vi "AB_Engine_Update_Paths_In_Palette_File.vi"(0 "old palette path":path, 1 "new palette path":path, 2 "old paths":path[](array[path]), 3 "new paths":path[](array[path]), 4 "old dir paths":path[](array[path]), 5 "new dir paths":path[](array[path]), 6 "application reference":refnum<vi>, 7 "error in":errorcluster) -> (19 "error out":errorcluster)   [LabVIEW 2020]
uses:
  <vilib>/Palette API/Palette Menu/Public Type Define/Palette Data.ctl
  <vilib>/Palette API/Palette Menu/Public Type Define/View Format.ctl
  <vilib>/Palette API/Palette Menu/Public Type Define/Items.ctl
  <vilib>/Palette API/Palette Menu/Public Type Define/Item.ctl
  <vilib>/Palette API/Palette Menu/Public Type Define/Help Info.ctl
  <vilib>/Palette API/Palette Menu/Public Type Define/Synchronize Info.ctl
  <vilib>/Palette API/Palette Menu/Public Type Define/Palette type.ctl
  <vilib>/Palette API/Palette Menu/Palette Menu.lvlib
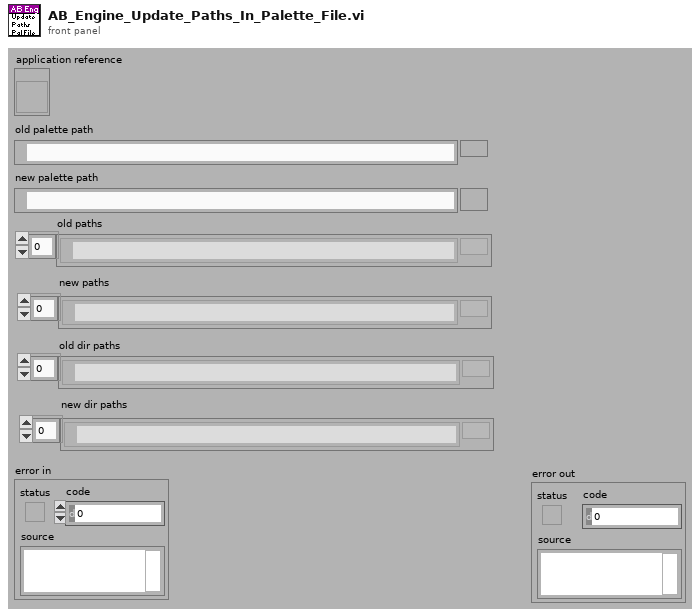
[diagram p1: front panel]
types:
  T1 = typedef "Palette Menu.lvlib/Palette Data.ctl" = cluster{"display name":string, "view format":T2, "palette width":i16, "items":T3, "256 color icon":picture, "B&W color icon":picture, "help information":T5, "palette description":string, "synchronize information":T6}
  T2 = typedef "Palette Menu.lvlib/View Format.ctl" = u16
  T3 = typedef "Palette Menu.lvlib/Items.ctl" = T4[]
  T4 = typedef "Palette Menu.lvlib/Item.ctl" = cluster{"item path":path, "library path":path, "use default lvlib palette":bool, "short name":string, "place VI contents":bool, "hide synchronized item":bool, "reserve spot for synch item":bool, "configure when placing VI contents":bool}
  T5 = typedef "Palette Menu.lvlib/Help Info.ctl" = cluster{"help tag":string, "help file path ":path}
  T6 = typedef "Palette Menu.lvlib/Synchronize Info.ctl" = cluster{"synchronize with directory":bool, "synchronize directory path":path}
  T7 = typedef "Palette Menu.lvlib/Palette type.ctl" = i32
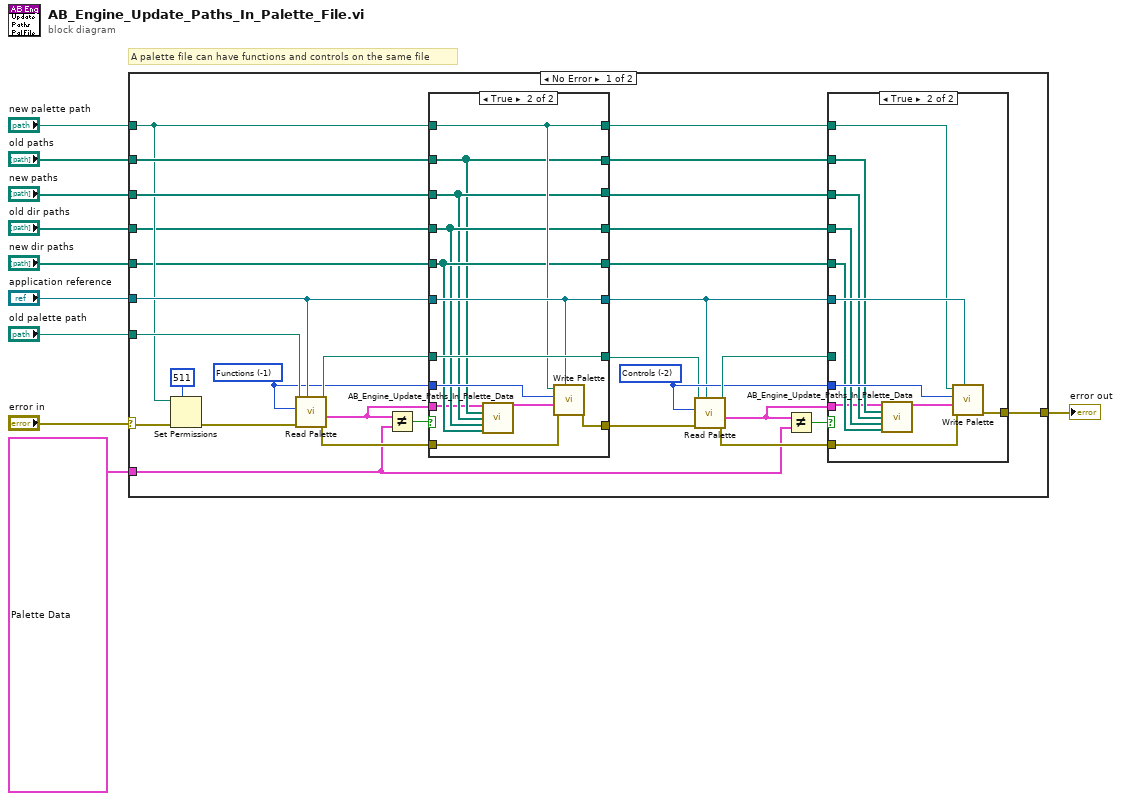
[diagram p0: block diagram]
diagram:
  # "A palette file can have functions and controls on the same file"
  n1 = case shown="No Error" "error in" {
    selector: "error in" -> [w18 w73]
    tunnel: "new palette path" -> [w15 _]
    tunnel: "old paths" -> [w35 _]
    tunnel: "new paths" -> [w34 _]
    tunnel: "application reference" -> [w33 _]
    tunnel: "old palette path" -> [w40 _]
    tunnel: [w19 w73] -> w4
    tunnel: T1 {"display name"="", "view format"=2, "palette width"=0, "items"=[], "256 color icon"=bytes[0], "B&W color icon"=bytes[0], "help information"={"help tag"="", "help file path "=path ""}, "palette description"="", "synchronize information"={"synchronize with directory"=FALSE, "synchronize directory path"=path ""}} ("palette data") -> [w20 _]
    tunnel: "old dir paths" -> [w14 _]
    tunnel: "new dir paths" -> [w13 _]
    frame No Error {
      w27 = T7 -2 items=["Functions"=-1, "Controls"=-2] ("palette type")
      w32 = T7 -1 items=["Functions"=-1, "Controls"=-2] ("palette type")
      n2 = Set Permissions(7:i16 511 ("permissions"), 8:w18, 11:w15) -> (0:w17:errorcluster)  [unwired: 2 in, 1 out]
      n3 = call <vilib>:"Read Palette.vi"("application reference"=w33, "error in (no error)"=w17, "palette type"=w32, "palette path"=w40) -> ("error out"=w38:errorcluster, "palette data"=w36:T1, "duplicate palette path"=w37:path)  [unwired: 5 in]
      n4 = Not Equal?(x=w36, y=w20) -> (x != y?=w39:bool)
      n5 = case shown="True" w39 {
        tunnel: w38 -> [w55 w71]
        tunnel: w37 -> [w56 w69]
        tunnel: w36 -> [_ w62]
        tunnel: w15 -> [w60 w67]
        tunnel: w35 -> [w59 w63]
        tunnel: w34 -> [w58 w64]
        tunnel: w33 -> [w57 w68]
        tunnel: w32 -> [_ w72]
        tunnel: [w55 w70] -> w26
        tunnel: [w56 w69] -> w25
        tunnel: [w57 w68] -> w24
        tunnel: [w58 w64] -> w23
        tunnel: [w59 w63] -> w22
        tunnel: [w60 w67] -> w21
        tunnel: [w54 w65] -> w12
        tunnel: w14 -> [w54 w65]
        tunnel: [w53 w66] -> w11
        tunnel: w13 -> [w53 w66]
        frame False {
        }
        frame True {
          n6 = call <vilib>:"AB_Engine_Update_Paths_In_Palette_Data.vi"("palette data in"=w62, "old paths"=w63, "new paths"=w64, "old dir paths"=w65, "new dir paths"=w66) -> ("palette data out"=w61:T1)  [unwired: 10 in]
          n7 = call <vilib>:"Write Palette.vi"("application reference"=w68, "error in (no error)"=w71, "palette data"=w61, "palette type"=w72, "palette path"=w67) -> ("error out"=w70:errorcluster)  [unwired: 6 in]
        }
      }
      n8 = call <vilib>:"Read Palette.vi"("application reference"=w24, "error in (no error)"=w26, "palette type"=w27, "palette path"=w25) -> ("error out"=w30:errorcluster, "palette data"=w28:T1, "duplicate palette path"=w29:path)  [unwired: 5 in]
      n9 = Not Equal?(x=w28, y=w20) -> (x != y?=w31:bool)
      n10 = case shown="True" w31 {
        tunnel: w30 -> [w41 w51]
        tunnel: w29 -> [_ _]
        tunnel: w28 -> [_ w43]
        tunnel: w21 -> [_ w48]
        tunnel: w22 -> [_ w44]
        tunnel: w23 -> [_ w45]
        tunnel: w24 -> [_ w49]
        tunnel: w27 -> [_ w52]
        tunnel: [w41 w50] -> w19
        tunnel: w12 -> [_ w46]
        tunnel: w11 -> [_ w47]
        frame False {
        }
        frame True {
          n11 = call <vilib>:"AB_Engine_Update_Paths_In_Palette_Data.vi"("palette data in"=w43, "old paths"=w44, "new paths"=w45, "old dir paths"=w46, "new dir paths"=w47) -> ("palette data out"=w42:T1)  [unwired: 10 in]
          n12 = call <vilib>:"Write Palette.vi"("application reference"=w49, "error in (no error)"=w51, "palette data"=w42, "palette type"=w52, "palette path"=w48) -> ("error out"=w50:errorcluster)  [unwired: 6 in]
        }
      }
    }
    frame Error {
    }
  }
  "error out" <- w4
